vi "S2C_SetLocalResults.vi"(8 "Error In":errorcluster, 11 "MenuRef":refnum<k9>) -> (0 "Error Out":errorcluster)   [LabVIEW 2015]
doc: "Toggles the \"Local File\" runtime menu item."
uses:
  Globals/S2C_Globals.vi
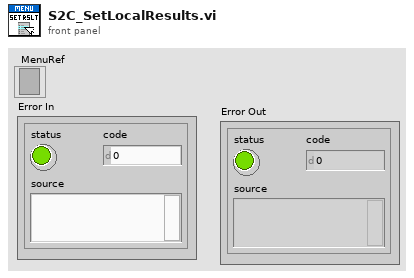
[diagram p1: front panel]
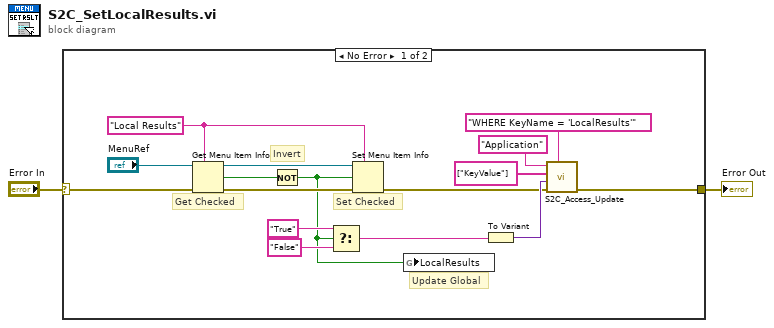
[diagram p0: block diagram]
diagram:
  n1 = case shown="No Error" "Error In" {
    selector: "Error In" -> [w18 w19]
    tunnel: [w4 w19] -> w1
    frame No Error {
      w16 = "Local Results" ("item tag")
      # "Update Global"
      # "Invert"
      # "Set Checked"
      # "Get Checked"
      n2 = Get Menu Item Info(7:w16, 8:w18, 11:"MenuRef") -> (0:w15:errorcluster, 3:w14:refnum<k9>, 4:w13:bool)  [unwired: 4 out]
      n3 = Not(x=w13) -> (.not. x?=w10:bool)
      n4 = Select(t="True", s=w10, f="False") -> (s? t:f=w3:string)
      n5 = Set Menu Item Info(6:w10, 7:w16, 8:w15, 11:w14) -> (0:w5:errorcluster)  [unwired: 3 in, 1 out]
      n6 = global write "S2C_Globals.vi" "LocalResults"(w10) -> ()
      n7 = To Variant(anything=w3) -> (Variant=w7:variant)
      n8 = call "S2C_Access_Update.vi"("Condition"="WHERE KeyName = 'LocalResults'", "Error In"=w5, "Data"=w7, "Columns"=string[] ["KeyValue"], "Table"="Application") -> ("Error Out"=w4:errorcluster)  [unwired: 6 in]
    }
    frame Error {
    }
  }
  "Error Out" <- w1
